vi "Digitizer Configure 1.vi"(7 "error in":errorcluster, 10 "Channel Parameters In":T1={"Channel Name"="0", "Number of Records"=0, "Reference Position"=0.0, "Minimum Record Length"=0, "Minimum Sample Rate"=0.0, "Maximum Input Frequency"=0.0, "Enforce Realtime"=FALSE, "Vertical Coupling"=enum."AC", "Probe Attenuation"=0.0, "Vertical Range (V)"=0.0, "Vertical Offset"=0.0, "Trigger Level"=0.0, "Trigger Type"=enum."Edge", "Trigger Source"=enum."Immediate", "Trigger Slope"=enum."Positive", "Digitizer 1 Used?"=FALSE, "Digitizer 1 Channels"="", "Digitizer 1 Reference"="", "Digitizer 1 Gain Multiplier"=nan, "Digitizer 2 Used?"=FALSE, "Digitizer 2 Channels"="", "Digitizer 2 Reference"="", "Session References"=[]}) -> (0 "error out":errorcluster, 3 "Channel Parameters Out":T1={"Channel Name"="0", "Number of Records"=0, "Reference Position"=0.0, "Minimum Record Length"=0, "Minimum Sample Rate"=0.0, "Maximum Input Frequency"=0.0, "Enforce Realtime"=FALSE, "Vertical Coupling"=enum."AC", "Probe Attenuation"=0.0, "Vertical Range (V)"=0.0, "Vertical Offset"=0.0, "Trigger Level"=0.0, "Trigger Type"=enum."Edge", "Trigger Source"=enum."Immediate", "Trigger Slope"=enum."Positive", "Digitizer 1 Used?"=FALSE, "Digitizer 1 Channels"="", "Digitizer 1 Reference"="", "Digitizer 1 Gain Multiplier"=nan, "Digitizer 2 Used?"=FALSE, "Digitizer 2 Channels"="", "Digitizer 2 Reference"="", "Session References"=[]})   [LabVIEW 2010]
uses:
  Typedef-Channel Parameters.ctl
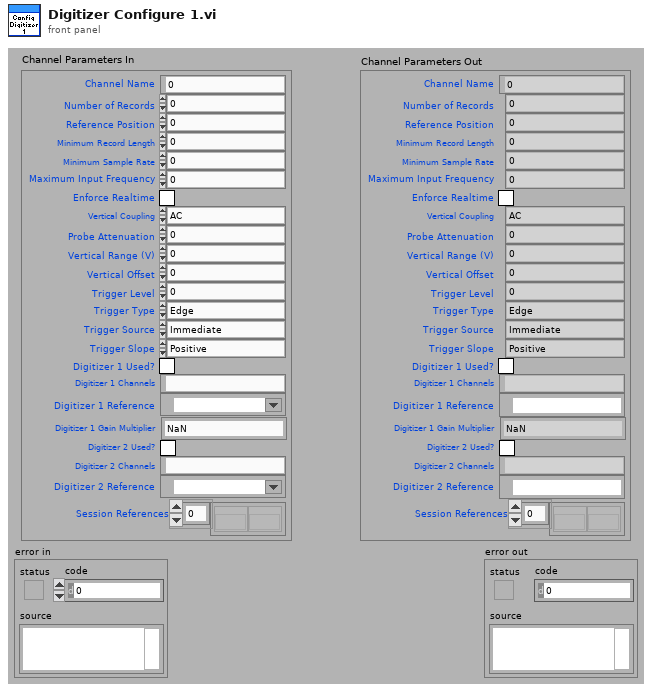
[diagram p1: front panel]
types:
  T1 = typedef "Typedef-Channel Parameters.ctl" = cluster{"Channel Name":string, "Number of Records":i32, "Reference Position":dbl, "Minimum Record Length":i32, "Minimum Sample Rate":dbl, "Maximum Input Frequency":dbl, "Enforce Realtime":bool, "Vertical Coupling":enum16{"AC", "DC", "Ground"}, "Probe Attenuation":dbl, "Vertical Range (V)":dbl, "Vertical Offset":dbl, "Trigger Level":dbl, "Trigger Type":enum16{"Edge", "Digital", "Immediate"}, "Trigger Source":enum16{"Immediate", "Channel 0", "Channel 1", "Channel 2", "Channel 3", "Channel 4", "Channel 5", "Channel 6", "Channel 7", "Extermal TRIG", "Software Trigger", "RTSI 0", "RTSI 1", "RTSI 2", "RTSI 3", "RTSI 4", "RTSI 5", "RTSI 6", "PF 0", "PF 1", "PF 2", "PXI Star Trigger"}, "Trigger Slope":enum16{"Positive", "Negative"}, "Digitizer 1 Used?":bool, "Digitizer 1 Channels":string, "Digitizer 1 Reference":refnum<k15>, "Digitizer 1 Gain Multiplier":dbl, "Digitizer 2 Used?":bool, "Digitizer 2 Channels":string, "Digitizer 2 Reference":refnum<k15>, "Session References":refnum<k20>[]}
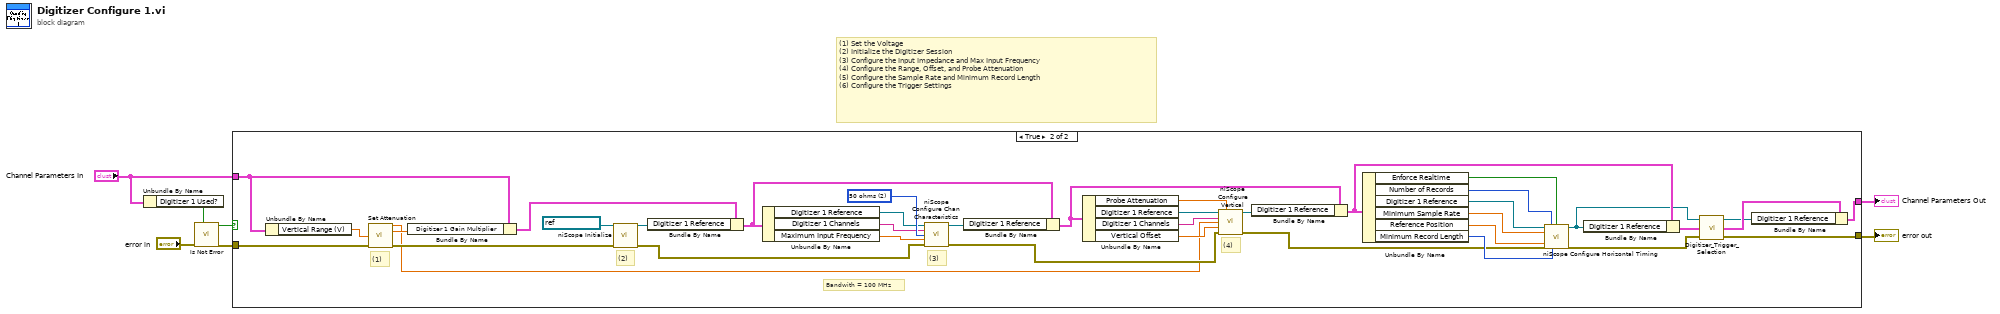
[diagram p0: block diagram]
diagram:
  # "(1) Set the Voltage\n(2) Initialize the Digitizer Session\n(3) Configure the Input Impedance and Max Input Frequency\n(4) Configure the Range, Offset, and Probe Attenuation\n(5) Configure the Sample Rate and Minimum Record Length \n(6) Configure the Trigger Settings"
  n1 = Unbundle By Name("Channel Parameters In") -> ("Digitizer 1 Used?"=w2:bool)
  n2 = call "Is Not Error.vi"("enable (T)"=w2, "error in"="error in") -> ("error out"=w3:errorcluster, "!error"=w1:bool)  [unwired: 4 in, 1 out]
  n3 = case shown="True" w1 {
    tunnel: [w9 w45] -> w7
    tunnel: "Channel Parameters In" -> [w8 w40]
    tunnel: [w8 w28] -> w6
    tunnel: w3 -> [w9 w44]
    frame False {
    }
    frame True {
      w21 = u32 2 items=["1 mega ohm"=0, "50 ohms"=2] ("input impedance")
      # "Bandwith = 100 MHz"
      # "(4)"
      # "(3)"
      # "(2)"
      # "(1)"
      n4 = Unbundle By Name(w40) -> ("Vertical Range (V)"=w43:dbl)
      n5 = call "Set Attenuation.vi"("vertical range"=w43, "error in"=w44) -> ("Requested Range"=w10:dbl, "Gain Multiplier"=w41:dbl, "error out"=w47:errorcluster)  [unwired: 11 in]
      n6 = Bundle By Name(cluster=w40, "Digitizer 1 Gain Multiplier"=w41) -> (w39:T1)
      n7 = call <instrlib>:"niScope Initialize.vi"("resource name"=refnum<k15> "PXI1Slot6", "error in"=w47) -> ("instrument handle"=w38:refnum<k15>, "error out"=w18:errorcluster)  [unwired: 12 in]
      n8 = Bundle By Name(cluster=w39, "Digitizer 1 Reference"=w38) -> (w17:T1)
      n9 = Unbundle By Name(w17) -> ("Digitizer 1 Reference"=w20:refnum<k15>, "Digitizer 1 Channels"=w19:string, "Maximum Input Frequency"=w22:dbl)
      n10 = call <instrlib>:"niScope Configure Chan Characteristics.vi"("instrument handle"=w20, "channels"=w19, "input impedance"=w21, "maximum input frequency"=w22, "error in"=w18) -> ("instrument handle out"=w16:refnum<k15>, "error out"=w15:errorcluster)  [unwired: 9 in]
      n11 = Bundle By Name(cluster=w17, "Digitizer 1 Reference"=w16) -> (w13:T1)
      n12 = Unbundle By Name(w13) -> ("Probe Attenuation"=w27:dbl, "Digitizer 1 Reference"=w36:refnum<k15>, "Digitizer 1 Channels"=w37:string, "Vertical Offset"=w11:dbl)
      n13 = call <instrlib>:"niScope Configure Vertical.vi"("instrument handle"=w36, "probe attenuation"=w27, "channels"=w37, "vertical range"=w10, "vertical offset"=w11, "error in"=w15) -> ("instrument handle out"=w12:refnum<k15>, "error out"=w14:errorcluster)  [unwired: 8 in]
      n14 = Bundle By Name(cluster=w13, "Digitizer 1 Reference"=w12) -> (w25:T1)
      n15 = Unbundle By Name(w25) -> ("Enforce Realtime"=w26:bool, "Number of Records"=w31:i32, "Digitizer 1 Reference"=w35:refnum<k15>, "Minimum Sample Rate"=w33:dbl, "Reference Position"=w34:dbl, "Minimum Record Length"=w32:i32)
      n16 = call <instrlib>:"niScope Configure Horizontal Timing.vi"("instrument handle"=w35, "number of records"=w31, "enforce realtime"=w26, "min sample rate"=w33, "reference position"=w34, "error in"=w14, "min record length"=w32) -> ("instrument handle out"=w23:refnum<k15>, "error out"=w46:errorcluster)  [unwired: 7 in]
      n17 = Bundle By Name(cluster=w25, "Digitizer 1 Reference"=w23) -> (w24:T1)
      n18 = call "Digitizer_Trigger_Selection.vi"("Error In"=w46, "Channel Parameters In"=w24, "instrument handle in"=w23) -> ("error out"=w45:errorcluster, "Channel Parameters Out"=w30:T1, "instrument handle out"=w29:refnum<k15>)
      n19 = Bundle By Name(cluster=w30, "Digitizer 1 Reference"=w29) -> (w28:T1)
    }
  }
  "error out" <- w7
  "Channel Parameters Out" <- w6
